vi "Parse JSON String (JSON).vi"(8 "error in (no error)":errorcluster, 11 "String":string) -> (0 "error out":errorcluster, 3 "Value":T1)   [LabVIEW 2015, in "JSON.lvlib"]
uses:
  JSON.lvlib
  JSON Value.ctl
  State.ctl
  Context.ctl
  Value.ctl
  Value Type.ctl
  Name-Value Pair.ctl
  Array Context.ctl
  Object Context.ctl
  <vilib>/regexp/Match Regular Expression.xnode
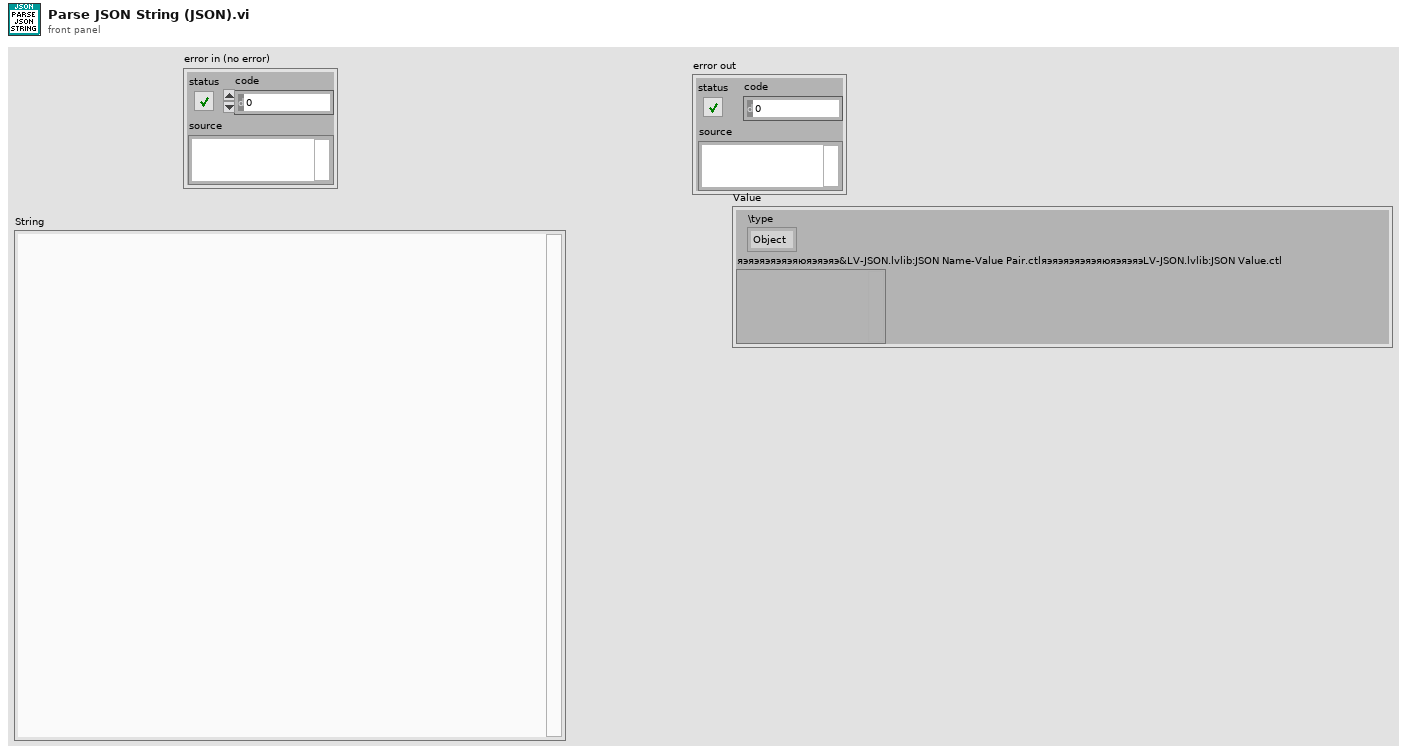
[diagram p1: front panel]
types:
  T1 = typedef "JSON.lvlib/JSON Value.ctl" = cluster{"\\type":enum16{"Object", "Array", "String", "Number", "Boolean", "Null"}, "яэяэяэяэяэяюяэяэяэ&LV-JSON.lvlib:JSON Name-Value Pair.ctlяэяэяэяэяэяюяэяэяэLV-JSON.lvlib:JSON Value.ctl":variant}
  T2 = typedef "JSON.lvlib/Value.ctl" = cluster{"Type":T3, "Value":variant}
  T3 = typedef "JSON.lvlib/Value Type.ctl" = enum16{"Object", "Array", "String", "Number", "Boolean", "Null"}
  T4 = typedef "JSON.lvlib/Context.ctl" = cluster{"Type":enum16{"Array", "Object", "Root"}, "Value":variant}
  T5 = typedef "JSON.lvlib/State.ctl" = enum16{"Value", "Object"}
  T6 = typedef "JSON.lvlib/Name-Value Pair.ctl" = cluster{"Name":string, "Value":T2}
  T7 = typedef "JSON.lvlib/Array Context.ctl" = cluster{"Array":T2[]}
  T8 = typedef "JSON.lvlib/Object Context.ctl" = cluster{"Object":T6[], "Key":string}
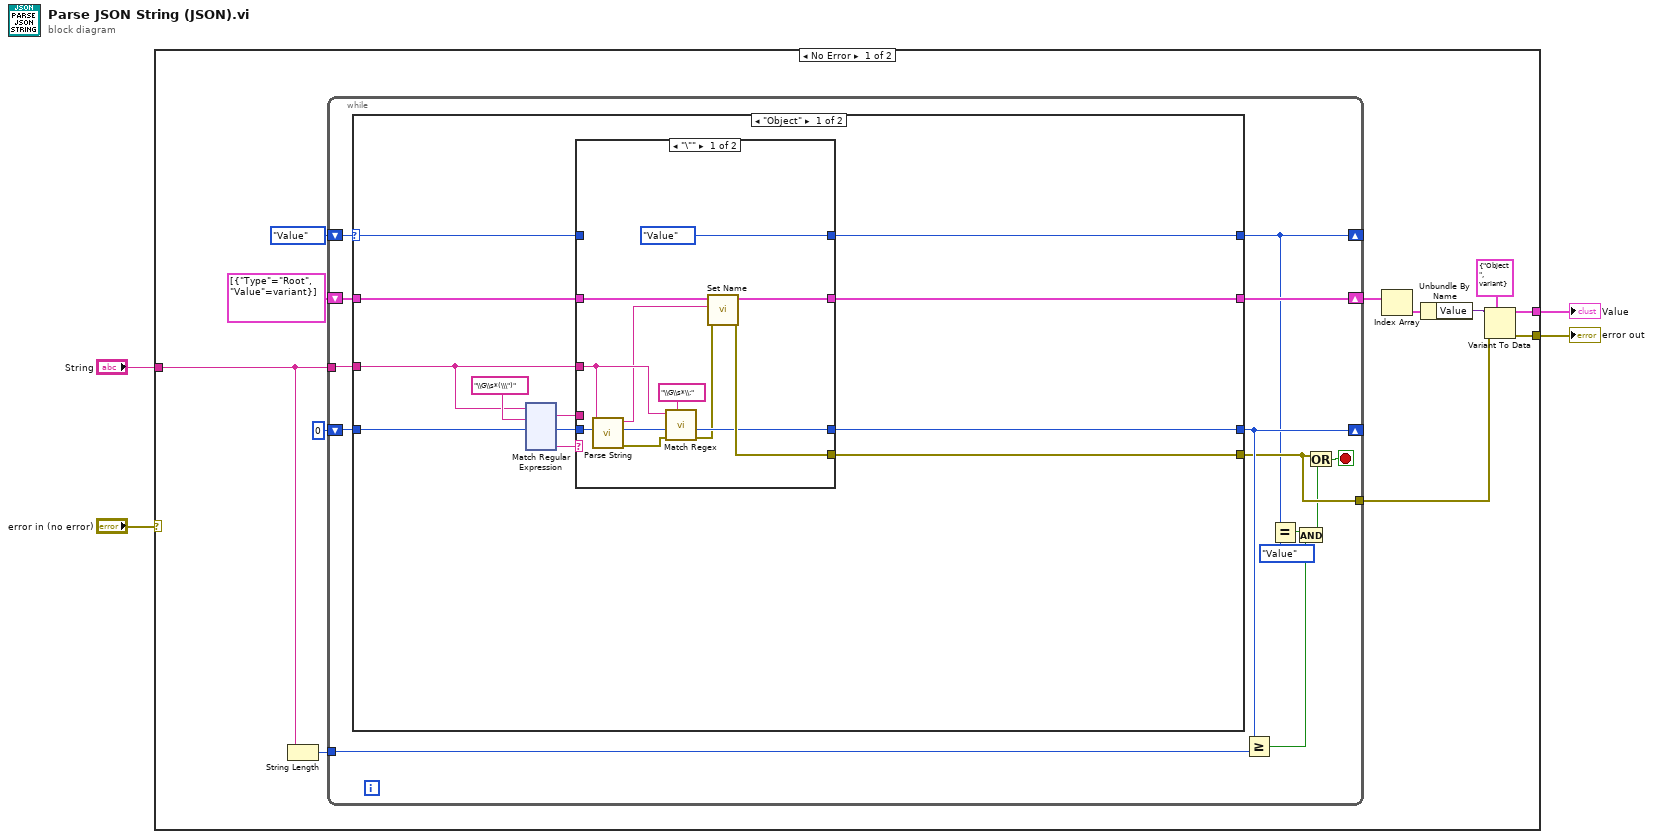
[diagram p0: block diagram]
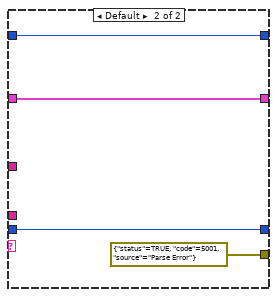
[diagram p2: hidden frame]
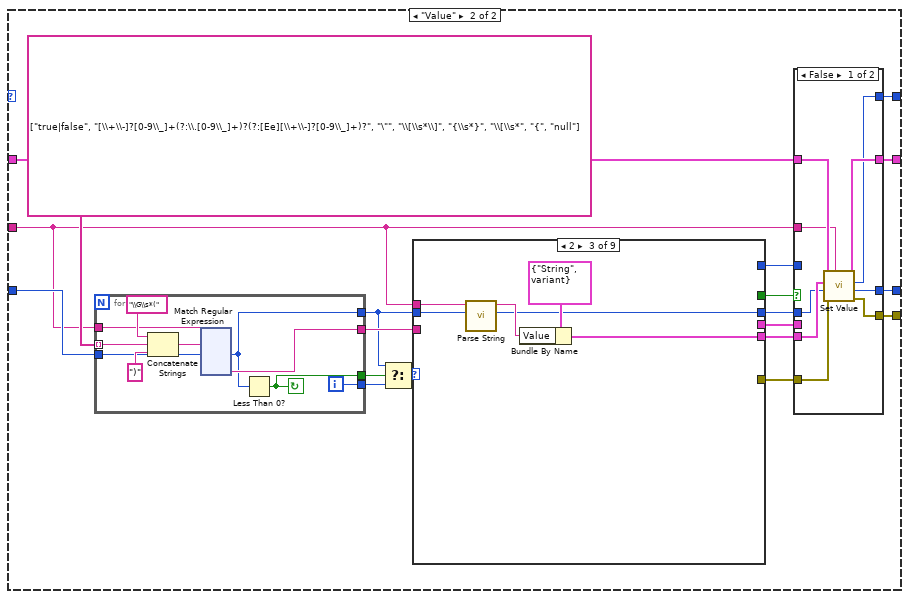
[diagram p3: hidden frame]
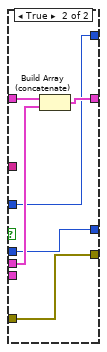
[diagram p4: hidden frame]
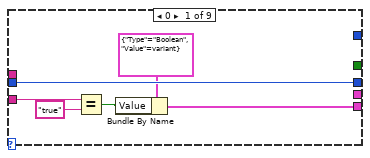
[diagram p5: hidden frame]
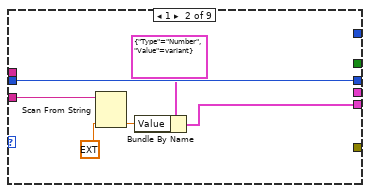
[diagram p6: hidden frame]
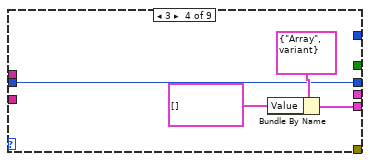
[diagram p7: hidden frame]
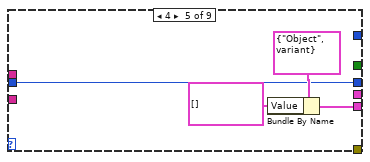
[diagram p8: hidden frame]
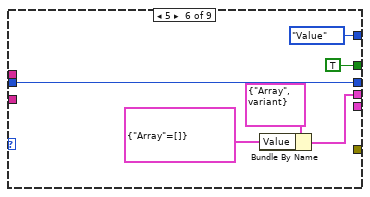
[diagram p9: hidden frame]
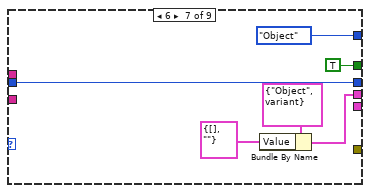
[diagram p10: hidden frame]
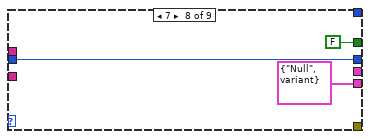
[diagram p11: hidden frame]
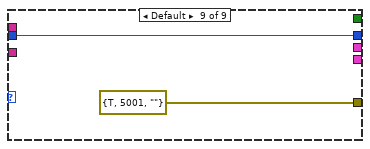
[diagram p12: hidden frame]
diagram:
  n1 = case shown="No Error" "error in (no error)" {
    selector: "error in (no error)" -> [_ w378]
    tunnel: "String" -> [w16 _]
    tunnel: [w14 _] -> w1
    tunnel: [w15 w378] -> w3
    frame No Error {
      n2 = String Length(string=w16) -> (length=w11:i32)
      n3 = while {
        tunnel: w16 -> [w29]
        shift-right: [w19] -> _
        shift-left: State."Value" ("State") -> [w30]
        shift-right: [w27] -> w7
        shift-left: T4[] [{"Type"=enum."Root", "Value"=variant}] ("Context out") -> [w26]
        shift-right: [w22] -> _
        shift-left: 0 -> [w28]
        tunnel: w11 -> [w24]
        tunnel: [w21] -> w8
        stop <- w25 stop-if-true
        n4 = case shown="\"Object\"" w30 {
          selector: w30 -> [w38 _]
          tunnel: w29 -> [w32 w175]
          tunnel: w28 -> [w31 w192]
          tunnel: [w39 w179] -> w19
          tunnel: [w37 w186] -> w27
          tunnel: w26 -> [w36 w185]
          tunnel: [w40 w176] -> w22
          tunnel: [w35 w183] -> w21
          frame "Object" {
            n5 = xnode "Match Regular Expression"("input string"=w32, "regular expression"="\\G\\s*(\\\")", "offset (0)"=w31) -> ("whole match"=w33:string, "offset past match"=w41:i32, "submatch 1"=w34:string)  [unwired: 3 in, 3 out]
            n6 = case shown="\"\\\"\"" w34 {
              tunnel: [w50 w57] -> w40
              tunnel: w41 -> [w47 w57]
              tunnel: [State."Value" ("State") w56] -> w39
              tunnel: w38 -> [_ w56]
              tunnel: [w51 w58] -> w37
              tunnel: w36 -> [w52 w58]
              tunnel: [w53 errorcluster {"status"=TRUE, "code"=5001, "source"="Parse Error"} ("error constant")] -> w35
              tunnel: w32 -> [w44 _]
              tunnel: w33 -> [_ _]
              frame "\"" {
                n7 = call "Parse String.vi"("start at"=w47, "TOML String"=w44) -> ("error out"=w45:errorcluster, "offset past match"=w46:i32, "String"=w43:string)  [unwired: 7 in]
                n8 = call "Match Regex.vi"("regular expression"="\\G\\s*\\:", "error in (no error)"=w45, "offset"=w46, "String"=w44) -> ("error out"=w48:errorcluster, "offset past match"=w50:i32)  [unwired: 4 in, 2 out]
                n9 = call "Set Name.vi"("error in (no error)"=w48, "Key"=w43, "Stack in"=w52) -> ("error out"=w53:errorcluster, "Stack out"=w51:T4[])  [unwired: 7 in]
              }
              frame Default {
              }
            }
          }
          frame "Value" {
            n10 = for {
              tunnel: string[] ["true|false", "[\\+\\-]?[0-9\\_]+(?:\\.[0-9\\_]+)?(?:[Ee][\\+\\-]?[0-9\\_]+)?", "\"", "\\[\\s*\\]", "{\\s*}", "\\[\\s*", "{", "null"] -> [w261] mode=indexing
              tunnel: w175 -> [w257]
              tunnel: w192 -> [w256]
              tunnel: [w255] -> w188
              tunnel: [w254] -> w187
              tunnel: [w253] -> w191
              tunnel: [w252] -> w190
              i -> [w252]
              stop <- w253 continue-if-true
              n11 = Concatenate Strings("\\G\\s*(" ("string"), w261, ")" ("string")) -> (w258:string)
              n12 = xnode "Match Regular Expression"("input string"=w257, "regular expression"=w258, "offset (0)"=w256) -> ("offset past match"=w254:i32, "submatch 1"=w255:string)  [unwired: 3 in, 4 out]
              n13 = Less Than 0?(x=w254) -> (x < 0?=w253:bool)
            }
            n14 = Select(t=w187, s=w191, f=w190) -> (s? t:f=w189:i32)
            n15 = case shown="2" w189 {
              tunnel: w188 -> [w213 w215 _ _ _ _ _ _ _]
              tunnel: w187 -> [w214 w220 w222 w228 w232 w240 w246 w249 w251]
              tunnel: [w214 w220 w221 w228 w232 w240 w246 w249 w251] -> w177
              tunnel: [_ _ _ _ _ _ _ _ errorcluster {"status"=TRUE, "code"=5001, "source"=""} ("error constant")] -> w184
              tunnel: [w209 w217 w225 w229 w233 _ _ T2 {"Type"=enum."Null", "Value"=variant} ("Value") _] -> w182
              tunnel: w175 -> [_ _ w224 _ _ _ _ _ _]
              tunnel: [_ _ _ _ _ TRUE TRUE FALSE _] -> w181
              tunnel: [_ _ _ _ _ w236 w243 _ _] -> w180
              tunnel: [_ _ _ _ _ State."Value" ("State") State."Object" ("State") _ _] -> w178
              frame 0 {
                n16 = Equal?(x=w213, y="true") -> (x = y?=w210:bool)
                n17 = Bundle By Name(cluster=T2 {"Type"=enum."Boolean", "Value"=variant} ("Value"), "Value"=w210) -> (w209:T2)
              }
              frame 1 {
                n18 = Scan From String(input string=w215, default 1=ext 0.0 ("default value 1")) -> (output 1=w218:ext)  [unwired: 3 in, 3 out]
                n19 = Bundle By Name(cluster=T2 {"Type"=enum."Number", "Value"=variant} ("Value"), "Value"=w218) -> (w217:T2)
              }
              frame 2 {
                n20 = call "Parse String.vi"("start at"=w222, "TOML String"=w224) -> ("offset past match"=w221:i32, "String"=w223:string)  [unwired: 7 in, 1 out]
                n21 = Bundle By Name(cluster=T2 {"Type"=enum."String", "Value"=variant} ("Value"), "Value"=w223) -> (w225:T2)
              }
              frame 3 {
                n22 = Bundle By Name(cluster=T2 {"Type"=enum."Array", "Value"=variant} ("Value"), "Value"=T2[] []) -> (w229:T2)
              }
              frame 4 {
                n23 = Bundle By Name(cluster=T2 {"Type"=enum."Object", "Value"=variant} ("Value"), "Value"=T6[] []) -> (w233:T2)
              }
              frame 5 {
                n24 = Bundle By Name(cluster=T4 {"Type"=enum."Array", "Value"=variant} ("Context"), "Value"=T7 {"Array"=[]} ("Array Context")) -> (w236:T4)
              }
              frame 6 {
                n25 = Bundle By Name(cluster=T4 {"Type"=enum."Object", "Value"=variant} ("Context"), "Value"=T8 {"Object"=[], "Key"=""} ("Table Context")) -> (w243:T4)
              }
              frame 7 {
              }
              frame Default {
              }
            }
            n26 = case shown="False" w181 {
              tunnel: [w202 w206] -> w186
              tunnel: w185 -> [w201 w207]
              tunnel: w184 -> [w200 w208]
              tunnel: [w199 w208] -> w183
              tunnel: w182 -> [w198 _]
              tunnel: w180 -> [_ w205]
              tunnel: [w197 w204] -> w179
              tunnel: w178 -> [_ w204]
              tunnel: w177 -> [w196 w203]
              tunnel: [w195 w203] -> w176
              tunnel: w175 -> [w194 _]
              frame False {
                n27 = call "Set Value.vi"("TOML string"=w194, "error in (no error)"=w200, "start position"=w196, "Value"=w198, "Values in"=w201) -> ("error out"=w199:errorcluster, "offset past match"=w195:i32, "State"=w197:T5, "Values out"=w202:T4[])  [unwired: 3 in]
              }
              frame True {
                n28 = Build Array (concatenate)(w207, w205) -> (w206:T4[])
              }
            }
          }
        }
        n29 = Greater Or Equal?(x=w22, y=w24) -> (x >= y?=w23:bool)
        n30 = Equal?(x=w19, y=State."Value") -> (x = y?=w17:bool)
        n31 = And(x=w17, y=w23) -> (x .and. y?=w20:bool)
        n32 = Or(x=w21, y=w20) -> (x .or. y?=w25:bool)
      }
      n33 = Index Array(array=w7) -> (element=w10:T4)  [unwired: 1 in]
      n34 = Unbundle By Name(w10) -> ("Value"=w9:variant)
      n35 = Variant To Data(error in=w8, type=T2 {"Type"=enum."Object", "Value"=variant} ("Value"), Variant=w9) -> (data=w14:T2, error out=w15:errorcluster)
    }
    frame Error {
    }
  }
  "error out" <- w3
  "Value" <- w1
